vi "default_config_OSC.vi"(0 "VISA resource in":refnum<visa-resource-name>="OSC", 11 "error in (no error)":errorcluster) -> (4 "VISA resource name out":refnum<visa-resource-name>, 15 "error out":errorcluster)   [LabVIEW 2011]
doc: "Sets OCS to its default settings for the chirped pulse measurement. The time base (time/div, sample rate, etc.) is not changed."
uses:
  <instrlib>/Tektronix 7000 Series/Public/Configure/Configure Trigger (Edge).vi
  <instrlib>/Tektronix 7000 Series/Tektronix 7000 Series.lvlib
panel:
  # "CH2 - Trigger Input Channel"
  # "CH1 - Microwave Input Channel"
  # "Resolution and Record Length"
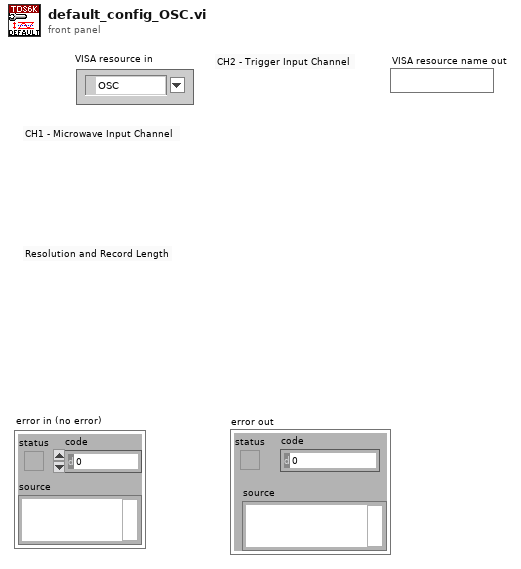
[diagram p1: front panel]
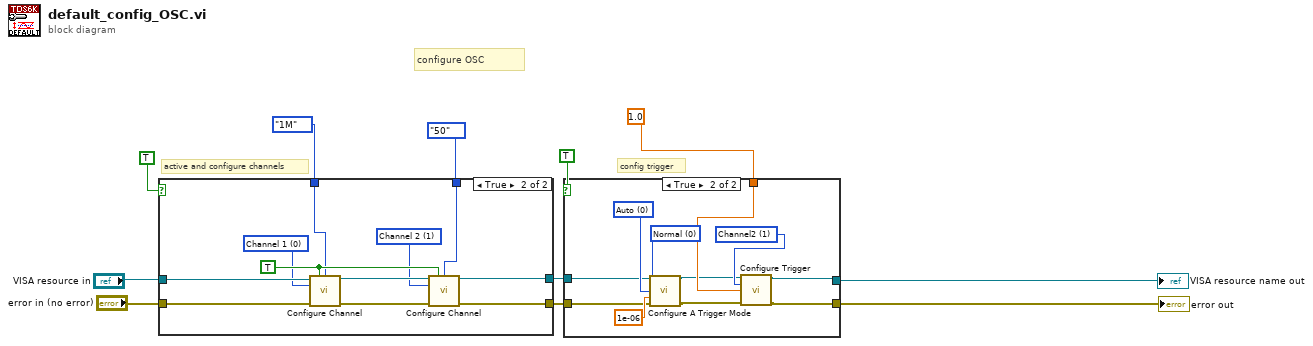
[diagram p0: block diagram]
diagram:
  # "config trigger"
  # "active and configure channels"
  # "configure OSC"
  n1 = case shown="True" TRUE ("channel") {
    tunnel: "VISA resource in" -> [w13 w22]
    tunnel: "error in (no error)" -> [w12 w21]
    tunnel: [w13 w20] -> w10
    tunnel: [w12 w19] -> w11
    tunnel: enum16{"1M", "50"}."50" ("CH2 Input Impedance") -> [_ w17]
    tunnel: enum16{"1M", "50"}."1M" ("CH1 Input Impedance") -> [_ w15]
    frame False {
    }
    frame True {
      w16 = u16 1 items=["Channel 1", "Channel 2", "Channel 3", "Channel 4", "Math 1", "Math 2", "Math 3", "Math 4", "Reference 1", "Reference 2", "Reference 3", "Reference 4"] ("Channel (0: Channel 1)")
      w18 = TRUE ("Enable Channel (T: Enable)")
      w14 = u16 0 items=["Channel 1", "Channel 2", "Channel 3", "Channel 4", "Math 1", "Math 2", "Math 3", "Math 4", "Reference 1", "Reference 2", "Reference 3", "Reference 4"] ("Channel (0: Channel 1)")
      n2 = call <instrlib>:"Configure Channel.vi"("VISA resource name"=w22, "Enable Channel (T: Enable)"=w18, "Input Impedance (0: 1M ohm)"=w15, "Channel (0: Channel 1)"=w14, "error in (no error)"=w21) -> ("VISA resource name out"=w23:refnum<visa-resource-name>, "error out"=w24:errorcluster)  [unwired: 9 in]
      n3 = call <instrlib>:"Configure Channel.vi"("VISA resource name"=w23, "Enable Channel (T: Enable)"=w18, "Input Impedance (0: 1M ohm)"=w17, "Channel (0: Channel 1)"=w16, "error in (no error)"=w24) -> ("VISA resource name out"=w20:refnum<visa-resource-name>, "error out"=w19:errorcluster)  [unwired: 9 in]
    }
  }
  n4 = case shown="True" TRUE ("trigger") {
    tunnel: w10 -> [w26 w29]
    tunnel: w11 -> [w25 w30]
    tunnel: [w26 w36] -> w2
    tunnel: [w25 w35] -> w1
    tunnel: 1.0 ("Trigger Level") -> [_ w34]
    frame False {
    }
    frame True {
      w31 = u16 0 items=["Normal", "Auto"] ("Trigger Mode (0:Normal)")
      w33 = u16 0 items=["Auto", "Time", "Random"] ("Holdoff Type (0:Auto)")
      w37 = u16 1 items=["Channel1"=0, "Channel2"=1, "Channel3"=2, "Channel4"=3, "Aux"=12, "Line"=13, "Digital Channel0"=14, "Digital Channel1"=15, "Digital Channel2"=16, "Digital Channel3"=17, "Digital Channel4"=18, "Digital Chennel5"=19, "Digital Channel6"=20, "Digital Channel7"=21, "Digital Channel8"=22, "Digital Channel9"=23, "Digital Channel10"=24, "Digital Channel11"=25, "Digital Channel12"=26, "Digital Channel13"=27, "Digital Channel14"=28, "Digital Channel15"=29] ("Trigger Channel")
      n5 = call <instrlib>:"Configure A Trigger Mode.vi"("VISA resource name"=w29, "Trigger Mode (0:Normal)"=w31, "Holdoff Type (0:Auto)"=w33, "Time Holdoff (1us)"=1e-06, "error in (no error)"=w30) -> ("VISA resource name out"=w28:refnum<visa-resource-name>, "error out"=w27:errorcluster)  [unwired: 9 in]
      n6 = call-poly <instrlib>:"Configure Trigger.vi"("VISA resource name"=w28, "Source (0:Channel1)"=w37, "Trigger Level (0.0V)"=w34, "error in (no error)"=w27) -> ("VISA resource name out"=w36:refnum<visa-resource-name>, "error out"=w35:errorcluster)  [unwired: 10 in]
    }
  }
  "VISA resource name out" <- w2
  "error out" <- w1
